vi "Write Start time.vi"(8 "error in (no error)":errorcluster, 10 "Start time":dbl, 11 "Timer in":refnum<class "Timer.lvclass">) -> (0 "error out":errorcluster, 3 "Timer out":refnum<class "Timer.lvclass">)   [LabVIEW 2019, in "Timer.lvclass"]
uses:
  Timer.lvclass
  Timer.lvclass/Timer.ctl
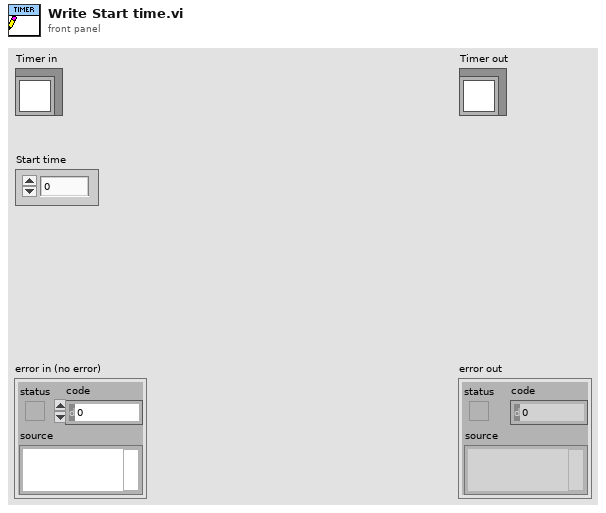
[diagram p1: front panel]
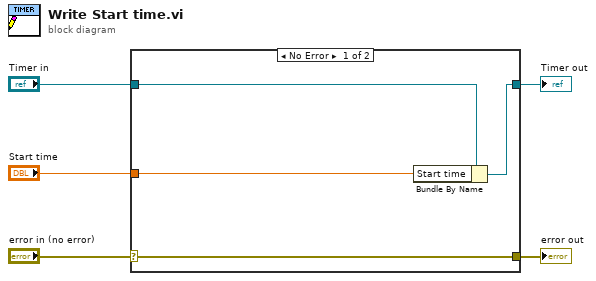
[diagram p0: block diagram]
diagram:
  n1 = case shown="No Error" "error in (no error)" {
    selector: "error in (no error)" -> [w9 w10]
    tunnel: [w9 w10] -> w4
    tunnel: [w7 w11] -> w2
    tunnel: "Timer in" -> [w8 w11]
    tunnel: "Start time" -> [w6 _]
    frame No Error {
      n2 = Bundle By Name(cluster=w8, "Start time"=w6) -> (w7:refnum<class "Timer.lvclass">)
    }
    frame Error {
    }
  }
  "error out" <- w4
  "Timer out" <- w2
